vi "Initialize.vi"(8 "error in (no error)":errorcluster, 10 "Input Angle (Deg.)":dbl) -> (0 "error out":errorcluster, 3 "Angle out":refnum<class "Angle.lvclass">)   [LabVIEW 2013, in "Angle.lvclass"]
doc: "Takes an inputted angle(deg.) double and creates an angle object"
uses:
  Angle.lvclass
  Angle.lvclass/Angle.ctl
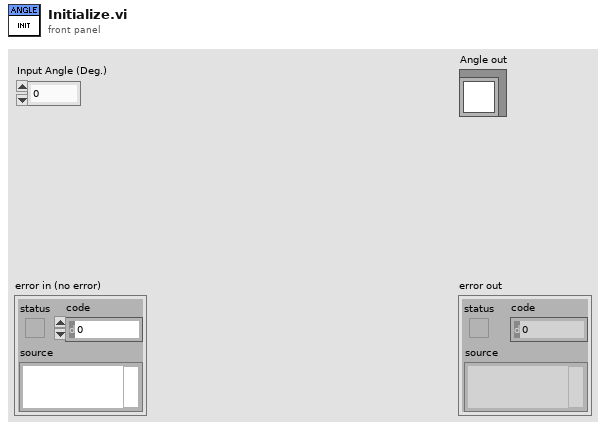
[diagram p1: front panel]
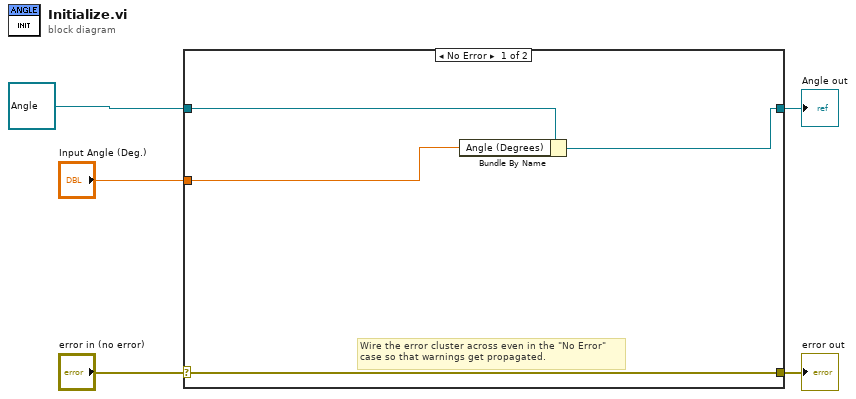
[diagram p0: block diagram]
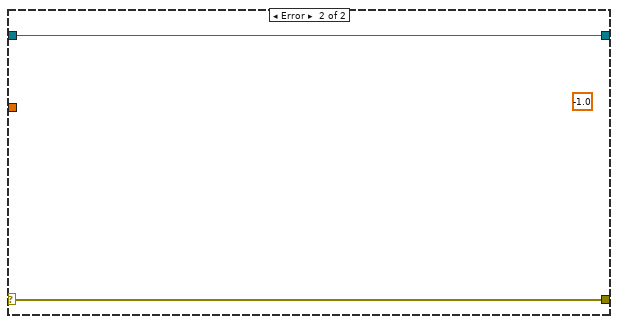
[diagram p2: hidden frame]
diagram:
  n1 = case shown="No Error" "error in (no error)" {
    selector: "error in (no error)" -> [w9 w11]
    tunnel: [w9 w11] -> w4
    tunnel: [w7 w10] -> w3
    tunnel: refnum<class "Angle.lvclass"> refnum ("Angle in") -> [w8 w10]
    tunnel: "Input Angle (Deg.)" -> [w6 _]
    frame No Error {
      # "Wire the error cluster across even in the \"No Error\"\ncase so that warnings get propagated."
      n2 = Bundle By Name(cluster=w8, "Angle (Degrees)"=w6) -> (w7:refnum<class "Angle.lvclass">)
    }
    frame Error {
      (unwired) -1.0 ("Input Angle (Deg.)")
    }
  }
  "error out" <- w4
  "Angle out" <- w3
